vi "Nack (SubVI).vi"   [LabVIEW 2019]
uses:
  <vilib>/rvi/eio/common/nirviEmuTemplateMethod_errors.vi
  <vilib>/eio/EIOMethodNode/EIOMethodNode.xnode
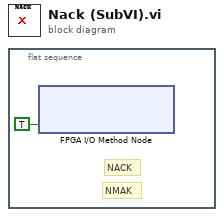
[diagram p0: block diagram]
diagram:
  n1 = flat-sequence {
    frame #0 {
      # "NMAK"
      # "NACK"
      n2 = xnode "FPGA I/O Method Node"("Enable"=TRUE) -> ()  [unwired: 1 in, 1 out]
    }
  }
